vi "_Destroy.vi"(8 "error in (no error)":errorcluster, 11 "DAQ Digital Code Scan in":refnum<class "DAQ Digital Code Scan.lvclass">) -> (0 "error out":errorcluster, 2 "finalized Scannable":refnum<class "Scannable.lvclass">)   [LabVIEW 2012, in "DAQ Digital Code Scan.lvclass"]
doc: "Release resources from and deallocate this Scanner instance."
uses:
  DAQ Digital Code Scan.lvclass
  Instruments/Utility Classes/Scannable/Scannable.lvclass
  LabVIEW-programs/Scanners/Scanner/Scanner.lvclass
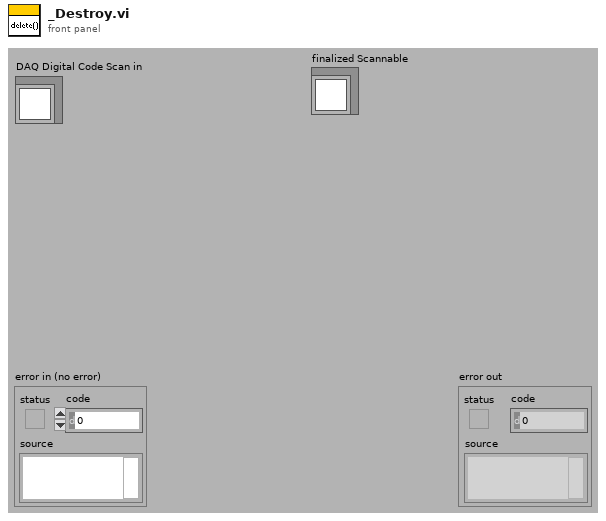
[diagram p1: front panel]
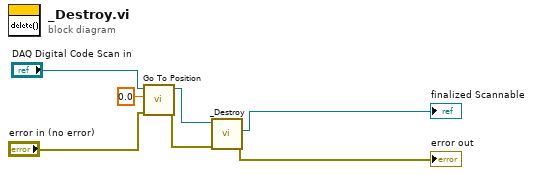
[diagram p0: block diagram]
diagram:
  n1 = call "Go To Position.vi"("error in (no error)"="error in (no error)", "Desired Position"=0.0, "DAQ Digital Code Scan in"="DAQ Digital Code Scan in") -> ("error out"=w1:errorcluster, "DAQ Digital Code Scan out"=w3:refnum<class "DAQ Digital Code Scan.lvclass">)  [unwired: 6 in, 1 out]
  n2 = call-parent "_Destroy.vi"("error in (no error)"=w1, "Scanner in"=w3) -> ("error out"=→"error out":errorcluster, "finalized Scannable"=→"finalized Scannable":refnum<class "Scannable.lvclass">)  [unwired: 8 in]
